vi "EditorSub createPictureMain.vi"(8 "error in (no error)":errorcluster, 11 "XY Graph":refnum<vi>) -> (0 "error out":errorcluster, 3 "2D Picture":picture)   [LabVIEW 2018]
panel:
  out "tempGraph":cluster{"X":dbl[], "Y":sgl[]}[](graph)
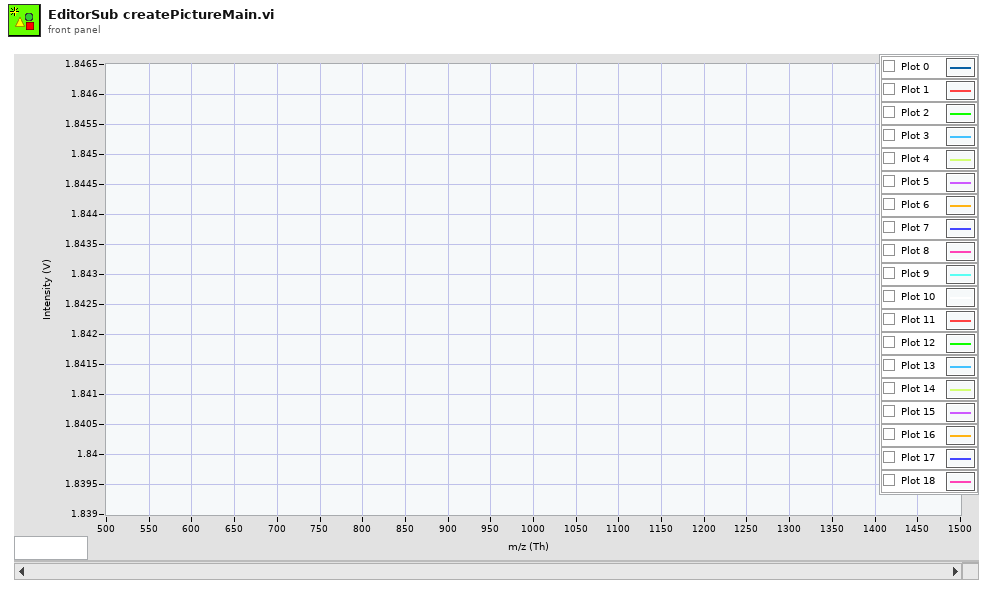
[diagram p1: front panel]
types:
  T1 = typedef "imagedata.ctl" = cluster{"image type":i32, "image depth":i32, "image":u8[], "mask":u8[], "colors":u32[], "Rectangle":cluster{"left":i16, "top":i16, "right":i16, "bottom":i16}}
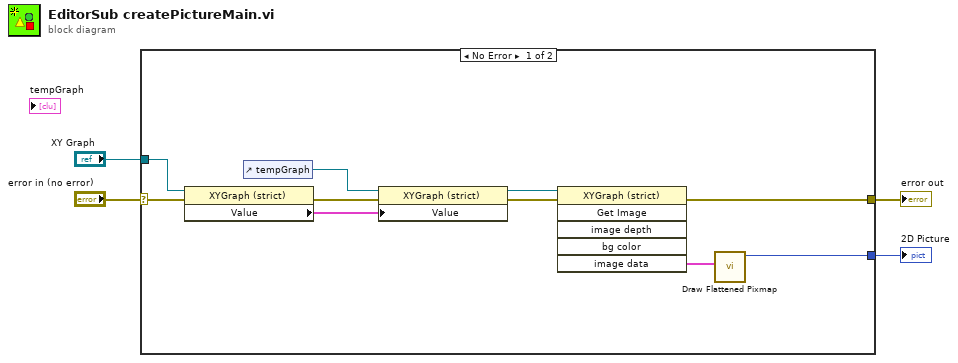
[diagram p0: block diagram]
diagram:
  n1 = case shown="No Error" "error in (no error)" {
    selector: "error in (no error)" -> [w8 w15]
    tunnel: "XY Graph" -> [w14 _]
    tunnel: [w9 _] -> w3
    tunnel: [w5 w15] -> w1
    frame No Error {
      n2 = property class="XYGraph (strict)"(reference=w14, error in=w8) -> (error out=w7:errorcluster, "Value"=w12:cluster{"X":dbl[], "Y":sgl[]}[])  [unwired: 1 out]
      n3 = control-ref of="tempGraph"() -> (w13:refnum<vi>)
      n4 = property class="XYGraph (strict)"(reference=w13, error in=w7, "Value"=w12) -> (reference out=w11:refnum<vi>, error out=w6:errorcluster)
      n5 = invoke class="XYGraph (strict)" method="Get Image"(reference=w11, error in=w6) -> (error out=w5:errorcluster, "image data"=w10:T1)  [unwired: 4 in, 4 out]
      n6 = call <vilib>:"Draw Flattened Pixmap.vi"("image data"=w10) -> ("new picture"=w9:picture)  [unwired: 8 in]
    }
    frame Error {
    }
  }
  "2D Picture" <- w3
  "error out" <- w1
